vi "Add Registered Process.vi"(6 "Process Runs (T)":bool=TRUE, 8 "error in (no error)":errorcluster, 9 "Process Name (Optional)":string, 10 "Process VI (Static VI Ref)":refnum<vi>, 11 "SMO":refnum<class "SMO.lvclass">) -> (0 "error out":errorcluster, 3 "SMO out":refnum<class "SMO.lvclass">)   [LabVIEW 2013, in "SMO.lvclass"]
doc: "---------------------------------------------------------------\nCopyright © 2014 JKI All rights reserved.\nAuthor: Philippe Guerit <philippe.guerit@jki.net>\nThis library is provided \"AS IS\" , WITHOUT WARRANTIES OR \nCONDITIONS OF ANY KIND, either express or implied.\nJKI. -- jki.net"
uses:
  SMO.lvclass
  SMO.lvclass/SMO.ctl
panel:
  # "For instructions on how to use the JKI State Machine Objects, examples and video tutorials, visit:\nhttp://jki.net/state-machine-objects/\n\nJKI State Machine Objects™\nhttp://jki.net/state-machine-objects/\nCopyright (C) 2005-2015, JKI <info@jki.net>\nALL RIGHTS RESERVED"
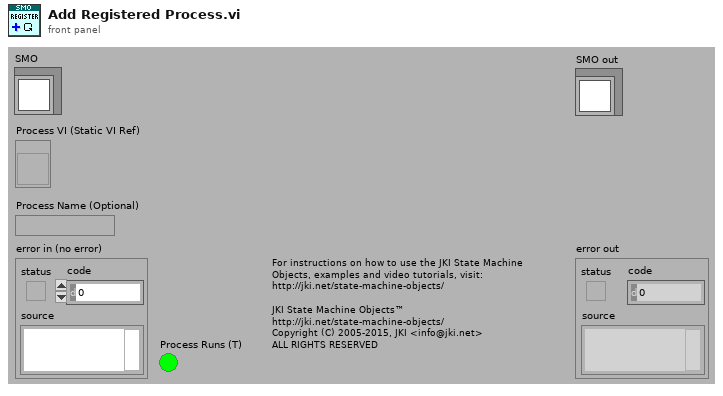
[diagram p1: front panel]
types:
  T1 = typedef "SMO.lvclass/PrivateData--Ref.ctl" = refnum<data-value>
  T2 = typedef "SMO.lvclass/PrivateData--Cluster.ctl" = cluster{"SMO Name":string, "Parent Call":T3, "Registered Processes":T4[], "Process Sync RendezVous":T5, "Process Error Notifier":refnum<notifier>, "Protected Events":T6, "Public Events":T7}
  T3 = typedef "SMO.lvclass/Parent Call--Enum.ctl" = enum16{"Allows parent to run", "Does not request parent to run"}
  T4 = typedef "SMO.lvclass/RegisteredProcessData--Cluster.ctl" = cluster{"Name":string, "Static VI Ref":refnum<vi>, "Running":bool}
  T5 = typedef "Rendezvous RefNum" = refnum<k1>
  T6 = typedef "SMO.lvclass/Protected Events.ctl" = cluster{"StopProcesses":refnum<user-event>, "AbortProcesses":refnum<user-event>}
  T7 = typedef "SMO.lvclass/Public Events.ctl" = cluster{"Error":refnum<user-event>}
  T8 = cluster{"Clone Name":string, "Process VI (Static VI Ref)":refnum<vi>, "Process Runs (T)":bool}
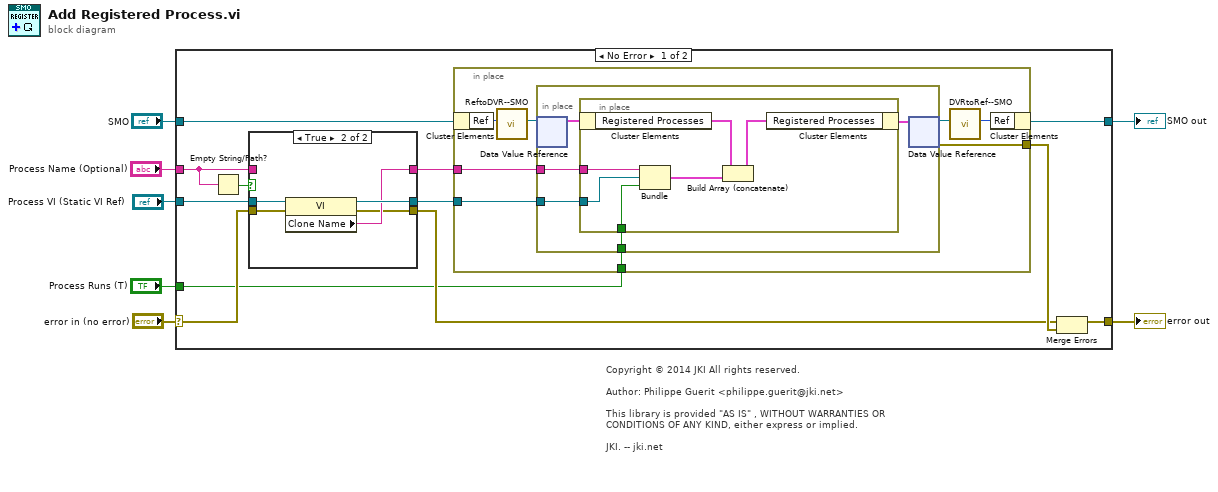
[diagram p0: block diagram]
diagram:
  # "Copyright © 2014 JKI All rights reserved.\n\nAuthor: Philippe Guerit <philippe.guerit@jki.net>\n\nThis library is provided \"AS IS\" , WITHOUT WARRANTIES OR \nCONDITIONS OF ANY KIND, either express or implied.\n\nJKI. -- jki.net"
  n1 = case shown="No Error" "error in (no error)" {
    selector: "error in (no error)" -> [w10 w48]
    tunnel: "Process VI (Static VI Ref)" -> [w15 _]
    tunnel: [w16 w48] -> w6
    tunnel: "Process Name (Optional)" -> [w11 _]
    tunnel: [w18 w47] -> w3
    tunnel: "SMO" -> [w19 w47]
    tunnel: "Process Runs (T)" -> [w8 _]
    frame No Error {
      n2 = Empty String/Path?(string/path=w11) -> (empty?=w13:bool)
      n3 = case shown="True" w13 {
        tunnel: w15 -> [w21 w27]
        tunnel: [w21 w26] -> w14
        tunnel: [w22 w25] -> w12
        tunnel: w11 -> [w22 _]
        tunnel: w10 -> [w20 w24]
        tunnel: [w20 w23] -> w9
        frame False {
        }
        frame True {
          n4 = property class="VI"(reference=w27, error in=w24) -> (reference out=w26:refnum<vi>, error out=w23:errorcluster, "Clone Name"=w25:string)
        }
      }
      n5 = in-place {
        in-place-border: w12 -> [w35]
        in-place-border: w14 -> [w34]
        in-place-border: [w33] -> w17
        in-place-border: w8 -> [w28]
        n6 = in-place-cluster #1(w19) -> ("Ref"=w32:u32)
        n7 = call "ReftoDVR--SMO.vi"("Ref"=w32) -> ("Ref"=w31:T1)  [unwired: 10 in]
        n8 = in-place {
          in-place-border: w35 -> [w39]
          in-place-border: w34 -> [w38]
          in-place-border: w28 -> [w36]
          n9 = in-place-dvr #2(w31) -> (w40:T2)  [unwired: 1 out]
          n10 = in-place {
            in-place-border: w39 -> [w44]
            in-place-border: w38 -> [w43]
            in-place-border: w36 -> [w41]
            n11 = in-place-cluster #3(w40) -> ("Registered Processes"=w46:T4[])
            n12 = Bundle("Clone Name"=w44, "Process VI (Static VI Ref)"=w43, "Process Runs (T)"=w41) -> (w42:T8)  [unwired: 1 in]
            n13 = Build Array (concatenate)(w46, w42) -> (w45:T4[])
            n14 = in-place-cluster #3("Registered Processes"=w45) -> (w37:T2)
          }
          n15 = in-place-dvr #2(w37) -> (w30:T1, w33:errorcluster)
        }
        n16 = call "DVRtoRef--SMO.vi"("Ref"=w30) -> ("Ref"=w29:u32)  [unwired: 10 in]
        n17 = in-place-cluster #1("Ref"=w29) -> (w18:refnum<class "SMO.lvclass">)
      }
      n18 = Merge Errors(w9, w17) -> (w16:errorcluster)
    }
    frame Error {
    }
  }
  "error out" <- w6
  "SMO out" <- w3
